vi "Stop Module.vi"(6 "Timeout to Wait for Stop (s) (-1: no timeout)":dbl=-1.0, 8 "error in":errorcluster, 9 "Wait for Module to Stop? (F)":bool, 10 "Origin":string) -> (0 "error out":errorcluster)   [LabVIEW 2023, in "Logger.lvlib"]
doc: "Send the Stop request to the Module's Main.vi.\n\nIf <b>Wait for Module to Stop?</b> is TRUE, this VI will wait until the module main VI stops, and will timeout at the <b>Timeout to Wait for Stop</b> value. This value defaults to \"-1\", which means the VI will not timeout, and will always wait until the module main VI stops before completing execution.\n\nNote: The <b>Timeout to Wait for Stop</b> value is ignored if 'Wait for Module to Stop?' is set to FALSE.\n_____\nBased on Delacor QMH Project Template 4.0.0.47.\n\n<b>Note:</b> This VI was modified by the <b>Validate DQMH Module</b> tool to add calls to the Semaphore VIs to synchronize actions between the Start Module and Stop Module VIs.\n_____\nBased on DQMH Project Template 6.1.0.94."
uses:
  Logger.lvlib
  Stop Argument--cluster.ctl
  <vilib>/event_ctls.llb/usereventprio.ctl
panel:
  # "Note: The 'Timeout to Wait for Stop' value is ignored if 'Wait for Module to Stop?' is set to FALSE."
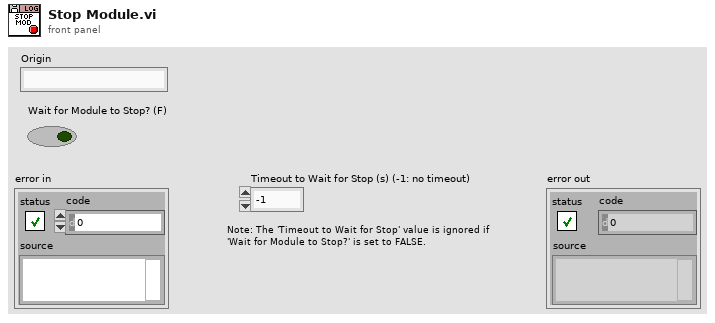
[diagram p1: front panel]
types:
  T1 = typedef "Logger.lvlib/Stop Argument--cluster.ctl" = cluster{"Origin":string, "Exit via Stop Module Req?":bool, "Wait for Module to stop?":bool}
  T2 = typedef "usereventprio.ctl" = enum32{"high priority", "normal priority"}
  T3 = typedef "Logger.lvlib/Request Events--cluster.ctl" = cluster{"Stop Module":refnum<user-event>, "Show Panel":refnum<user-event>, "Hide Panel":refnum<user-event>, "Get Module Execution Status":refnum<user-event>, "Show Diagram":refnum<user-event>, "Stop Logging":refnum<user-event>, "Log Data":refnum<user-event>, "Initialize File":refnum<user-event>}
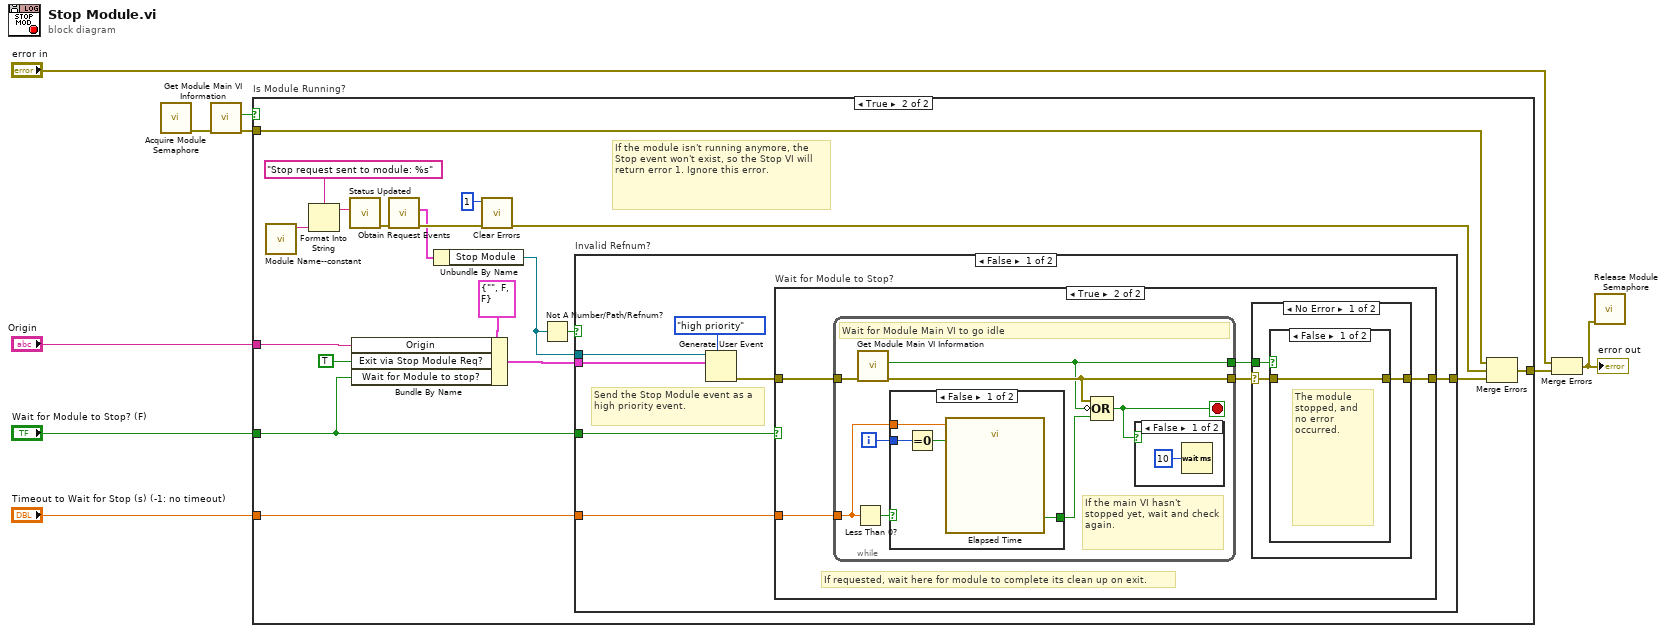
[diagram p0: block diagram]
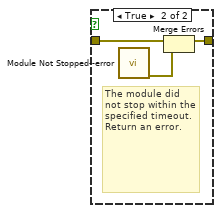
[diagram p4: hidden frame]
diagram:
  n1 = call "Acquire Module Semaphore.vi"() -> ("error out"=w1:errorcluster)  [unwired: 11 in]
  n2 = call "Get Module Main VI Information.vi"("error in"=w1) -> ("error out"=w7:errorcluster, "Is Module Running?"=w6:bool)  [unwired: 7 in, 2 out]
  n3 = case "Is Module Running?" shown="True" w6 {
    tunnel: [w10 w28] -> w4
    tunnel: "Origin" -> [_ w27]
    tunnel: w7 -> [w10 w16]
    tunnel: "Wait for Module to Stop? (F)" -> [_ w12]
    tunnel: "Timeout to Wait for Stop (s) (-1: no timeout)" -> [_ w11]
    frame False {
      # "The module is not running, there is no need to run the Stop Module code."
    }
    frame True {
      # "If the module isn't running anymore, the Stop event won't exist, so the Stop VI will return error 1. Ignore this error."
      n4 = call "Module Name--constant.vi"() -> ("Module Name"=w23:string)  [unwired: 11 in]
      n5 = Format Into String(format string="Stop request sent to module: %s", w23) -> (resulting string=w24:string)  [unwired: 2 in, 1 out]
      n6 = call "Status Updated.vi"("Status"=w24) -> ("error out"=w15:errorcluster)  [unwired: 10 in]
      n7 = Bundle By Name(cluster=T1 {"Origin"="", "Exit via Stop Module Req?"=FALSE, "Wait for Module to stop?"=FALSE} ("event data"), "Origin"=w27, "Exit via Stop Module Req?"=TRUE, "Wait for Module to stop?"=w12) -> (w19:T1)
      n8 = call "Obtain Request Events.vi"("error in (no error)"=w15) -> ("error out"=w29:errorcluster, "Logger Request Events"=w26:T3)  [unwired: 9 in]
      n9 = Unbundle By Name(w26) -> ("Stop Module"=w20:refnum<user-event>)
      n10 = call <vilib>:"Clear Errors.vi"("error in (no error)"=w29, "specific error code to clear (0: all)"=1) -> ("error out"=w14:errorcluster)  [unwired: 4 in, 1 out]
      n11 = Not A Number/Path/Refnum?(number/path/refnum=w20) -> (NaN/Path/Refnum?=w21:bool)
      n12 = case "Invalid Refnum?" shown="False" w21 {
        tunnel: [w31 _] -> w18
        tunnel: w20 -> [w36 _]
        tunnel: w19 -> [w34 _]
        tunnel: w12 -> [w32 _]
        tunnel: w11 -> [w30 _]
        frame False {
          # "Send the Stop Module event as a high priority event."
          n13 = Generate User Event(priority (normal)=usereventprio."high priority", user event=w36, event data cluster=w34) -> (error out=w33:errorcluster)  [unwired: 1 in, 1 out]
          n14 = case "Wait for Module to Stop?" shown="True" w32 {
            tunnel: w33 -> [w37 w41]
            tunnel: [w37 w39] -> w31
            tunnel: w30 -> [_ w42]
            frame False {
            }
            frame True {
              # "If requested, wait here for module to complete its clean up on exit."
              n15 = while {
                tunnel: w42 -> [w53]
                tunnel: w41 -> [w57]
                tunnel: [w56] -> w40
                tunnel: [w55] -> w38
                i -> [w58]
                stop <- w51 stop-if-true
                # "If the main VI hasn't stopped yet, wait and check again."
                # "Wait for Module Main VI to go idle"
                n16 = Less Than 0?(x=w53) -> (x < 0?=w52:bool)
                n17 = call "Get Module Main VI Information.vi"("error in"=w57) -> ("error out"=w56:errorcluster, "Is Module Running?"=w55:bool)  [unwired: 7 in, 2 out]
                n18 = case shown="False" w52 {
                  tunnel: w53 -> [w60 _]
                  tunnel: w58 -> [w62 _]
                  tunnel: [w61 _] -> w54
                  frame False {
                    n19 = Equal To 0?(x=w62) -> (x = 0?=w63:bool)
                    n20 = call "Elapsed Time"("Time Target (s)"=w60, "Reset"=w63) -> ("Time has Elapsed"=w61:bool)  [unwired: 10 in, 7 out]
                  }
                  frame True {
                    # "User specified a timeout of -1, so don't keep track of the elapsed time since this loop started."
                  }
                }
                n21 = Compound Arithmetic op=OR(w56, invert w55, w54) -> (w51:bool)
                n22 = case shown="False" w51 {
                  frame False {
                    n23 = Wait (ms)(milliseconds to wait=u32 10) -> ()  [unwired: 1 out]
                  }
                  frame True {
                  }
                }
              }
              n24 = case shown="No Error" w40 {
                selector: w40 -> [w44 w50]
                tunnel: [w43 w50] -> w39
                tunnel: w38 -> [w45 _]
                frame No Error {
                  n25 = case shown="False" w45 {
                    tunnel: w44 -> [w46 w49]
                    tunnel: [w46 w48] -> w43
                    frame False {
                      # "The module stopped, and no error occurred."
                    }
                    frame True {
                      # "The module did not stop within the specified timeout. Return an error."
                      n26 = call "Module Not Stopped--error.vi"() -> ("error out"=w47:errorcluster)  [unwired: 11 in]
                      n27 = Merge Errors(w49, w47) -> (w48:errorcluster)
                    }
                  }
                }
                frame Error {
                  # "An error occurred while waiting for the module to stop. Return that error."
                }
              }
            }
          }
        }
        frame True {
          # "Module is exiting. No need to send the standard \"not running\" error that is sent in other request VIs."
        }
      }
      n28 = Merge Errors(w16, w14, w18) -> (w28:errorcluster)
    }
  }
  n29 = Merge Errors("error in", w4) -> (w3:errorcluster)
  "error out" <- w3
  n30 = call "Release Module Semaphore.vi"("error in"=w3) -> ()  [unwired: 10 in, 1 out]
